vi "Main.vi"() -> ()   [LabVIEW 2013]
panel:
  in  "stop":bool
  out "Karta do akwizycji danych":bool
  out "Uk³ad pomiarowy":bool
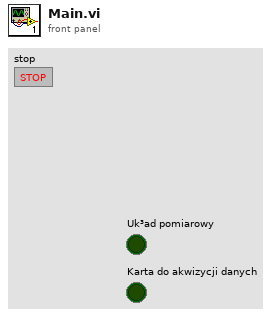
[diagram p1: front panel]
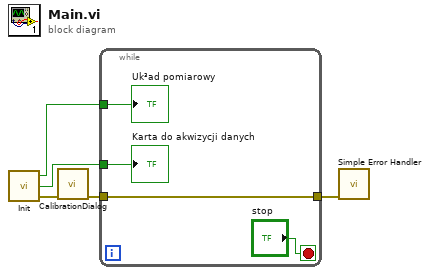
[diagram p0: block diagram]
diagram:
  n1 = call "Init.vi"() -> ("error out"=w2:errorcluster, "DAQ"=w4:bool, "Servo"=w3:bool)  [unwired: 3 in]
  n2 = call "CalibrationDialog.vi"("error in"=w2) -> ("error out"=w1:errorcluster)  [unwired: 5 in, 1 out]
  n3 = while {
    tunnel: w1 -> [w9]
    tunnel: [w9] -> w5
    tunnel: w3 -> [w8]
    tunnel: w4 -> [w7]
    stop <- "stop" stop-if-true
    "Uk³ad pomiarowy" <- w8
    "Karta do akwizycji danych" <- w7
  }
  n4 = call <vilib>:"Simple Error Handler.vi"("error in (no error)"=w5) -> ()  [unwired: 4 in, 5 out]
